vi "General Polynomial Fit Coefficients (Bisquare).vi"(0 "Y":dbl[](array[numeric]), 1 "polynomial order":i32=2, 2 "Coefficient Constraint":cluster{"order":i32, "coefficient":dbl}[](array[cluster]), 5 "X":dbl[](array[numeric]), 7 "Weight":dbl[](array[numeric]), 9 "tolerance":dbl=0.0001, 13 "algorithm":T1 items=["SVD", "Givens", "Givens2", "Householder", "LU Decomposition", "Cholesky", "SVD for Rank Deficient H"]) -> (4 "Polynomial Coefficients":dbl[](array[numeric]), 15 "error":i32)   [LabVIEW 2014, in "NI_AALPro.lvlib"]
uses:
  NI_AALPro.lvlib
  General Linear Fit Algorithm.ctl
  lvanlys.dll
panel:
  # "Bisquare General Polynomial Fit Coefficients"
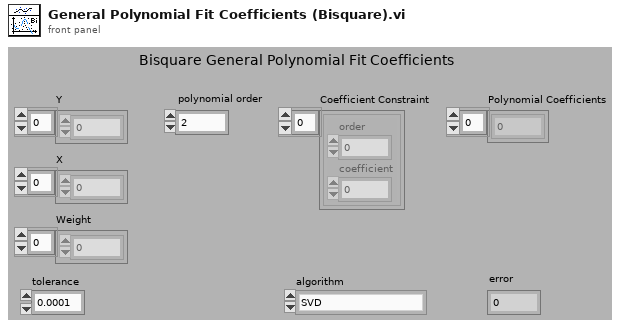
[diagram p1: front panel]
types:
  T1 = typedef "NI_AALPro.lvlib/General Linear Fit Algorithm.ctl" = u16
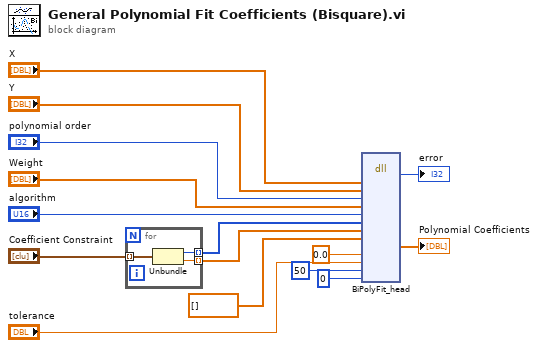
[diagram p0: block diagram]
diagram:
  n1 = for {
    tunnel: "Coefficient Constraint" -> [w18] mode=indexing
    tunnel: [w17] -> w15 mode=indexing
    tunnel: [w16] -> w14 mode=indexing
    n2 = Unbundle(w18) -> ("order"=w17:i32, "coefficient"=w16:dbl)
  }
  n3 = dll-call lib="C:/Program Files (x86)/National Instruments/LabVIEW 2014/resource/lvanlys.*" fn="BiPolyFit_head"("xH"="X", "yH"="Y", "Order"="polynomial order", "weightH"="Weight", "algorithm"="algorithm", "specOrderH"=w15, "specCoefH"=w14, "BestFitH"=dbl[] [], "mse"=0.0, "tolerance"="tolerance", "maxIter"=50, "iscoef"=0) -> ("return type"=→"error":i32, "CoefH"=→"Polynomial Coefficients":dbl[])  [unwired: 12 in, 6 out]
